vi "Parse Data Object Simple.vi"(8 "x":i32, 11 "Data":T1(array[cluster])) -> (0 "ROI 1, Frame 1, Row 1":dbl[](graph), 3 "ROI 1, Frame 1":dbl[][](graph))   [LabVIEW 2015, in "LightField Automation.lvclass"]
uses:
  LightField Automation.lvclass
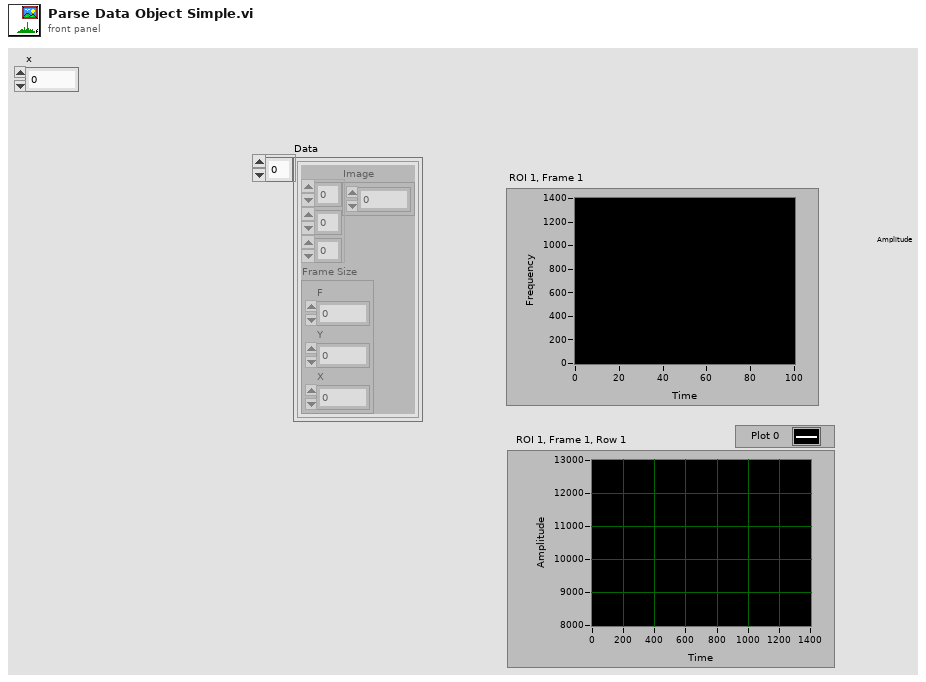
[diagram p1: front panel]
types:
  T1 = cluster{"Image":dbl[][][], "Frame Size":cluster{"F":i32, "Y":i32, "X":i32}}[]
  T2 = cluster{"Image":dbl[][][], "Frame Size":cluster{"F":i32, "Y":i32, "X":i32}}
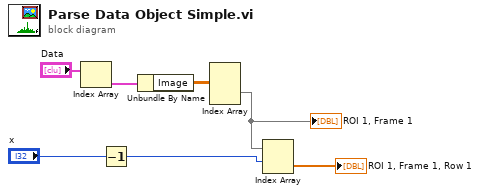
[diagram p0: block diagram]
diagram:
  n1 = Index Array(array="Data") -> (element=w7:T2)  [unwired: 1 in]
  n2 = Decrement(x="x") -> (x-1=w2:i32)
  n3 = Unbundle By Name(w7) -> ("Image"=w6:dbl[][][])
  n4 = Index Array(array=w6) -> (element=w5:dbl[][])  [unwired: 3 in]
  "ROI 1, Frame 1" <- w5
  n5 = Index Array(array=w5, index (row)=w2) -> (element=→"ROI 1, Frame 1, Row 1":dbl[])  [unwired: 1 in]
